vi "Get Latest Values.vi"(0 "reference in":refnum<class "NI-DAQmx.lvclass">, 5 "error in (no error)":errorcluster) -> (14 "reference out":refnum<class "NI-DAQmx.lvclass">, 15 "Latest Values":dbl[](array[numeric]), 16 "Signal List":T1[](array[typedef]), 19 "error out":errorcluster)   [LabVIEW 2018, in "NI-DAQmx.lvclass"]
uses:
  NI-DAQmx.lvclass
  controls/IO Signal List.ctl
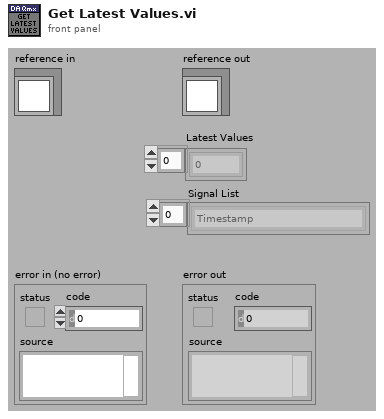
[diagram p1: front panel]
types:
  T1 = typedef "IO Signal List.ctl" = enum16{"Timestamp", "PSU_FB_U_VDC", "PSU_FB_I_AMP", "PSU_FB_W_WATT", "PSU_CMD_U_VDC", "PSU_CMD_I_AMP", "PSU_CMD_OUTPUT", "LCR_PRIMARY", "LCR_SECONDARY", "UV_R_mOhm", "UW_R_mOhm", "VW_R_mOhm", "UV_L_µH", "UW_L_µH", "VW_L_µH", "U_U_VDC", "V_U_VDC", "W_U_VDC", "U_I_AMP", "V_I_AMP", "W_I_AMP", "PWM_CMD_DC_%", "PWM_CMD_VDC", "PWM_CMD_Hz", "PWM_FB_DC_%", "PWM_FB_VDC", "PWM_FB_Hz", "DO_RELAY_U_LCR_A", "DO_RELAY_V_LCR_A", "DO_RELAY_V_LCR_B", "DO_RELAY_W_LCR_B", "DIFF_UV_UW_L_µH", "DIFF_UV_VW_L_µH", "DIFF_UW_VW_L_µH", "DIFF_UV_UW_R_mOhm", "DIFF_UV_VW_R_mOhm", "DIFF_UW_VW_R_mOhm", "DIFF_UV_U_VDC", "DIFF_UW_U_VDC", "DIFF_VW_U_VDC"}
  T2 = typedef "NI-DAQmx.lvclass/ObjectAttributes.ctl" = cluster{"AI Task":refnum<k21>, "DO Task":refnum<k21>, "AO Task":refnum<k21>, "Latest Values":dbl[], "Signal List":T1[], "PWM Duty Cycle (%)":dbl, "PWM Amplitude (V)":dbl, "PWM Frequency (Hz)":dbl, "DO States":bool[]}
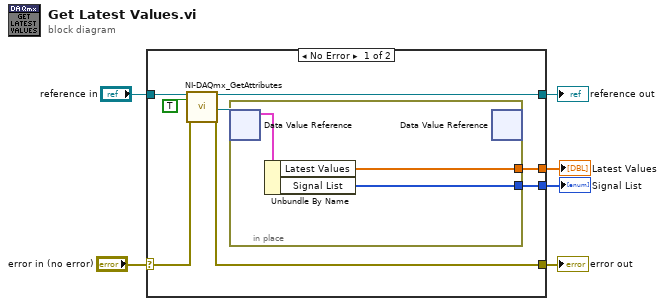
[diagram p0: block diagram]
diagram:
  n1 = case shown="No Error" "error in (no error)" {
    selector: "error in (no error)" -> [w14 w19]
    tunnel: [w13 w19] -> w5
    tunnel: [w11 w18] -> w3
    tunnel: "reference in" -> [w12 w18]
    tunnel: [w8 _] -> w2
    tunnel: [w7 _] -> w1
    frame No Error {
      n2 = call "NI-DAQmx_GetAttributes.vi"("reference in"=w12, "OnlyGetDvrReference(False)"=TRUE, "error in (no error)"=w14) -> ("reference out"=w11:refnum<class "NI-DAQmx.lvclass">, "DataRef"=w10:refnum<data-value>, "error out"=w13:errorcluster)  [unwired: 13 in, 1 out]
      n3 = in-place {
        in-place-border: [w17] -> w8
        in-place-border: [w15] -> w7
        n4 = in-place-dvr #1(w10) -> (w16:T2)  [unwired: 1 out]
        n5 = Unbundle By Name(w16) -> ("Latest Values"=w17:dbl[], "Signal List"=w15:T1[])
        n6 = in-place-dvr #1() -> ()  [unwired: 1 in, 2 out]
      }
    }
    frame Error {
    }
  }
  "error out" <- w5
  "reference out" <- w3
  "Latest Values" <- w2
  "Signal List" <- w1
